vi "Analytical Model.vi"() -> ()   [LabVIEW 2019]
uses:
  <vilib>/addons/Control Design/_Model Construction/Model Typedefs.llb/CD State Space Model (MIMO).ctl
  <vilib>/addons/Control Design/_Model Construction/Model Typedefs.llb/CD General Elements.ctl
  <vilib>/addons/Control Design/_Model Construction/Data Typedefs.llb/CD Time Info.ctl
  <vilib>/addons/Control Design/_Model Construction/Model Creation.llb/Model Creation SubVI/cd_Create Symbolic State Space Model.vi
  <vilib>/addons/Control Design/_Time Response Analysis/Time Response.llb/Time Response subVI/cd_Step Response (State-Space).vi
  <vilib>/addons/Control Design/_Model Construction/NI_LinSys_Model Creation.lvlib
  <vilib>/addons/Control Design/_Time Response Analysis/NI_CD_Time Response.lvlib
  <vilib>/addons/Control Design/_Model Construction/NI_LinSys_Data Typedefs.lvlib
  <vilib>/addons/Control Design/_Model Construction/NI_LinSys_Model Typedefs.lvlib
panel:
  out "Step Response Graph":cluster{"time":dbl[], dbl[]}[](graph)
  in  "Symbolic D":string[][](array[string])=[["0"]]
  in  "Symbolic C":string[][](array[string])=[["1"]]
  in  "Symbolic B":string[][](array[string])=[["G*kt/(R*J)"]]
  in  "Symbolic A":string[][](array[string])=[["-G^2*kt/(kv*R*J)"]]
  in  "Variables":cluster{"Name":string, " Value":dbl}[](array[cluster])=[{"Name"="m", " Value"=10.0}, {"Name"="b", " Value"=20.0}, {"Name"="k", " Value"=50.0}] {"Value" format="%.2f"}
  out "State Space Model":T1 {"Transport Delay" format="%.2f"; "D" format="%#.2g"; "C" format="%#.2g"; "B" format="%#.2g"; "A" format="%#.2g"; "properties"."Sampling Time" format="%#.6p"; "properties"."Output Delays" format="%.4f"; "properties"."Input Delays" format="%.4f"}
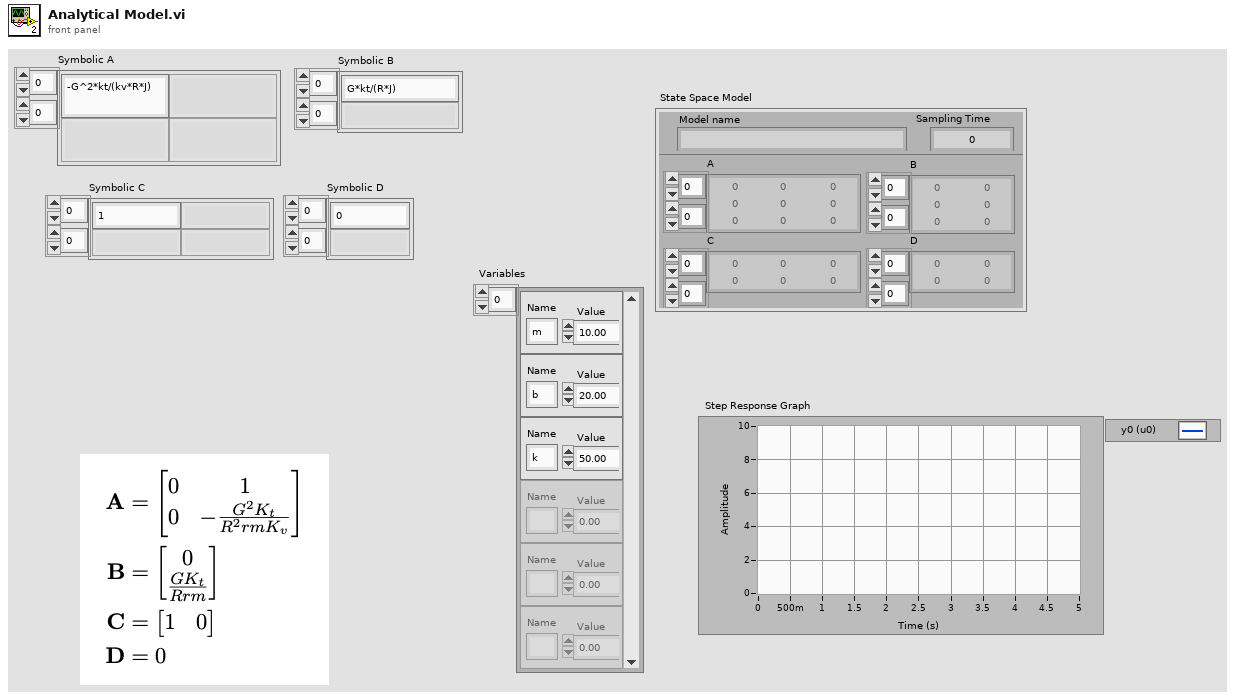
[diagram p1: front panel]
types:
  T1 = typedef "NI_LinSys_Model Typedefs.lvlib/CD State Space Model (MIMO).ctl" = cluster{"properties":T2, "A":dbl[][], "B":dbl[][], "C":dbl[][], "D":dbl[][], "StateNames":string[], "Transport Delay":dbl[][]}
  T2 = typedef "NI_LinSys_Model Typedefs.lvlib/CD General Elements.ctl" = cluster{"Model name":string, "Input names":string[], "Output names":string[], "Input Delays":dbl[], "Output Delays":dbl[], "Sampling Time":dbl, "Notes":string}
  T3 = typedef "NI_LinSys_Data Typedefs.lvlib/CD Time Info.ctl" = cluster{"t0":dbl, "dt":dbl, "tf":dbl}
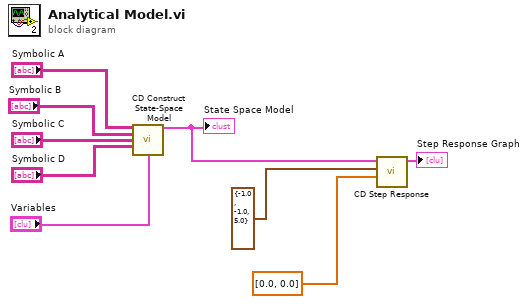
[diagram p0: block diagram]
diagram:
  n1 = call-poly <vilib>:"CD Construct State-Space Model.vi"("Symbolic A"="Symbolic A", "Symbolic B"="Symbolic B", "Symbolic C"="Symbolic C", "Symbolic D"="Symbolic D", "Variables"="Variables") -> ("State Space Model"=w1:T1)  [unwired: 9 in, 1 out]
  "State Space Model" <- w1
  n2 = call-poly <vilib>:"CD Step Response.vi"("Initial Conditions"=dbl[] [0.0, 0.0], "Time Range"=T3 {"t0"=-1.0, "dt"=-1.0, "tf"=5.0}, "State-Space Model"=w1) -> ("Step Response Graph"=→"Step Response Graph":cluster{"time":dbl[], dbl[]}[])  [unwired: 5 in, 3 out]
